vi "遥控参数对话框.vi"() -> (2 "遥控参数选择输出":T1(ring), 3 "确定?":bool)   [LabVIEW 2016, in "环境动力监测库.lvlib" / "空调库.lvlib"]
panel:
  in  "取消":bool
  in  "确定":bool
  in  "遥控参数选择":T1(ring)
  # "遥控参数选择"
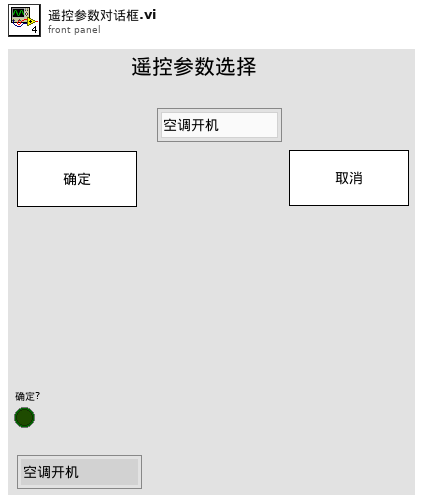
[diagram p1: front panel]
types:
  T1 = enum16{"空调开机", "空调关机", "制冷开启", "制冷关闭", "制热开启", "制热关闭"}
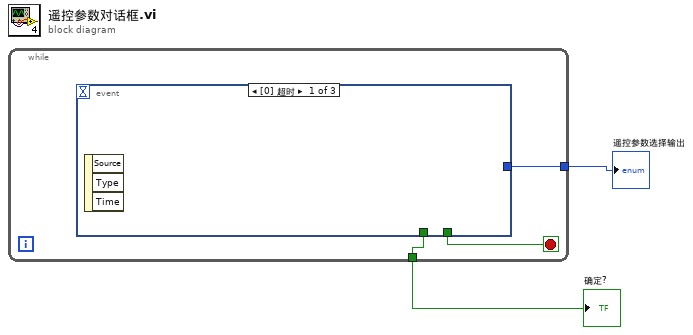
[diagram p0: block diagram]
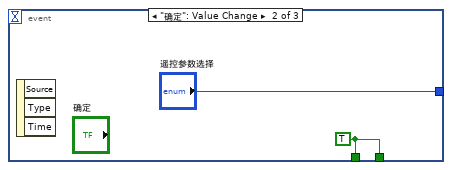
[diagram p2: hidden frame]
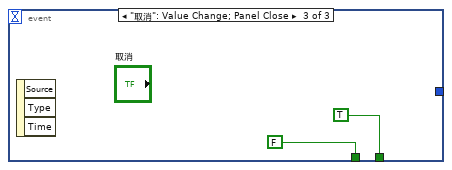
[diagram p3: hidden frame]
diagram:
  n1 = while {
    tunnel: [w5] -> w2
    tunnel: [w3] -> w1
    stop <- w4 stop-if-true
    n2 = event shown="[0] 超时" {
      selector: _ -> [_ _ _]
      dyn-events: _ -> [_ _ _]
      timeout: _ -> [_ _ _]
      tunnel: [_ w6 TRUE] -> w4
      tunnel: [_ "遥控参数选择" _] -> w5
      tunnel: [_ w6 FALSE] -> w3
      event Timeout {
        n3 = event-data() -> ()  [unwired: 1 in, 3 out]
      }
      event "确定": Value Change {
        w6 = TRUE
        n4 = event-data() -> ()  [unwired: 1 in, 3 out]
      }
      event "取消": Value Change; Panel Close {
        n5 = event-data() -> ()  [unwired: 1 in, 3 out]
      }
    }
  }
  "确定?" <- w1
  "遥控参数选择输出" <- w2
